vi "http parse header string.vi"(11 "raw string":string) -> (0 "no field name":bool, 1 "no crlf":bool, 2 "header field data":string, 3 "header field name":string, 5 "continuation":bool)   [LabVIEW 2016, in "Basic HTTP server.lvclass"]
uses:
  Basic HTTP server.lvclass
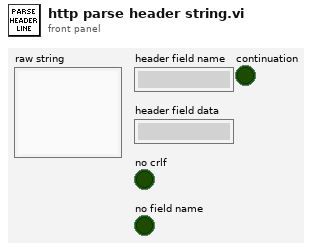
[diagram p1: front panel]
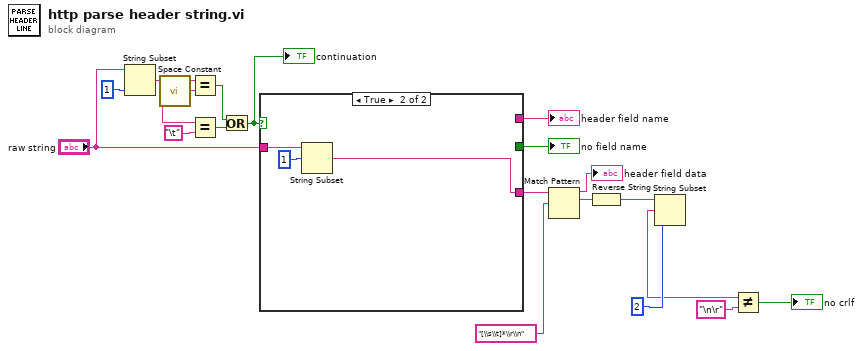
[diagram p0: block diagram]
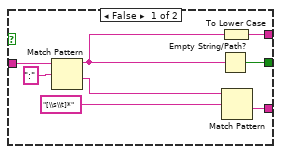
[diagram p2: hidden frame]
diagram:
  n1 = String Subset(string="raw string", length (rest)=1 ("length (rest)")) -> (substring=w11:string)  [unwired: 1 in]
  n2 = call <vilib>:"Space Constant.vi"() -> ("String"=w10:string)
  n3 = Equal?(x=w11, y=w10) -> (x = y?=w15:bool)
  n4 = Equal?(x=w11, y="\t") -> (x = y?=w14:bool)
  n5 = Or(x=w15, y=w14) -> (x .or. y?=w1:bool)
  "continuation" <- w1
  n6 = case shown="True" w1 {
    tunnel: [w27 _] -> w18
    tunnel: "raw string" -> [w26 w30]
    tunnel: [w25 _] -> w13
    tunnel: [w24 w28] -> w7
    frame False {
      n7 = Match Pattern(string=w26, regular expression=":") -> (before substring=w20:string, after substring=w22:string)  [unwired: 1 in, 2 out]
      n8 = Empty String/Path?(string/path=w20) -> (empty?=w27:bool)
      n9 = To Lower Case(string=w20) -> (all lower case string=w25:string)
      n10 = Match Pattern(string=w22, regular expression="[\\s\\t]*") -> (after substring=w24:string)  [unwired: 1 in, 3 out]
    }
    frame True {
      n11 = String Subset(string=w30, offset (0)=1) -> (substring=w28:string)  [unwired: 1 in]
    }
  }
  "no field name" <- w18
  "header field name" <- w13
  n12 = Match Pattern(string=w7, regular expression="[\\s\\t]*\\r\\n") -> (before substring=→"header field data":string, match substring=w6:string)  [unwired: 1 in, 2 out]
  n13 = Reverse String(1:w6) -> (0:w5:string)
  n14 = String Subset(string=w5, length (rest)=2 ("length (rest)")) -> (substring=w3:string)  [unwired: 1 in]
  n15 = Not Equal?(x=w3, y="\n\r" ("regular expression")) -> (x != y?=→"no crlf":bool)
